vi "使用范例_多列数据存储.vi"() -> ()   [LabVIEW 2020]
panel:
  in  "y2":dbl[](array[numeric])=[1.0, 0.9951847266721969, 0.9807852804032304, 0.9569403357322088, 0.9238795325112867, 0.881921264348355, 0.8314696123025452, 0.773010453362737, 0.7071067811865476, 0.6343932841636455, 0.5555702330196023, 0.4713967368259978, 0.38268343236508984, 0.29028467725446233, 0.19509032201612833, 0.09801714032956077, 6.123233995736766e-17, -0.09801714032956065, -0.1950903220161282, -0.29028467725446216, -0.3826834323650897, -0.4713967368259977, -0.555570233019602, -0.6343932841636454, -0.7071067811865475, -0.773010453362737, -0.8314696123025453, -0.8819212643483549, -0.9238795325112867, -0.9569403357322088, -0.9807852804032304, -0.9951847266721968, -1.0, -0.9951847266721969, -0.9807852804032304, -0.9569403357322089, -0.9238795325112868, -0.881921264348355, -0.8314696123025455, -0.7730104533627371, -0.7071067811865477, -0.6343932841636459, -0.5555702330196022, -0.47139673682599786, -0.38268343236509034, -0.29028467725446244, -0.19509032201612866, -0.09801714032956045, -1.8369701987210297e-16, 0.09801714032956009, 0.1950903220161283, 0.29028467725446205, 0.38268343236509, 0.4713967368259976, 0.5555702330196018, 0.6343932841636456, 0.7071067811865474, 0.7730104533627367, 0.8314696123025452, 0.8819212643483548, 0.9238795325112865, 0.9569403357322088, 0.9807852804032303, 0.9951847266721969, 1.0]
  in  "x":dbl[](array[numeric])=[0.0, 0.09817477042468103, 0.19634954084936207, 0.2945243112740431, 0.39269908169872414, 0.4908738521234052, 0.5890486225480862, 0.6872233929727672, 0.7853981633974483, 0.8835729338221293, 0.9817477042468103, 1.0799224746714913, 1.1780972450961724, 1.2762720155208536, 1.3744467859455345, 1.4726215563702154, 1.5707963267948966, 1.6689710972195777, 1.7671458676442586, 1.8653206380689396, 1.9634954084936207, 2.061670178918302, 2.1598449493429825, 2.2580197197676637, 2.356194490192345, 2.454369260617026, 2.552544031041707, 2.650718801466388, 2.748893571891069, 2.84706834231575, 2.945243112740431, 3.043417883165112, 3.141592653589793, 3.2397674240144743, 3.3379421944391554, 3.436116964863836, 3.5342917352885173, 3.6324665057131984, 3.730641276137879, 3.8288160465625602, 3.9269908169872414, 4.025165587411922, 4.123340357836604, 4.221515128261284, 4.319689898685965, 4.417864669110647, 4.516039439535327, 4.614214209960009, 4.71238898038469, 4.81056375080937, 4.908738521234052, 5.006913291658733, 5.105088062083414, 5.203262832508095, 5.301437602932776, 5.399612373357457, 5.497787143782138, 5.595961914206819, 5.6941366846315, 5.792311455056181, 5.890486225480862, 5.988660995905543, 6.086835766330224, 6.1850105367549055, 6.283185307179586]
  in  "y1":dbl[](array[numeric])=[0.0, 0.0980171403295606, 0.19509032201612825, 0.29028467725446233, 0.3826834323650898, 0.47139673682599764, 0.5555702330196022, 0.6343932841636455, 0.7071067811865475, 0.773010453362737, 0.8314696123025452, 0.8819212643483549, 0.9238795325112867, 0.9569403357322089, 0.9807852804032304, 0.9951847266721968, 1.0, 0.9951847266721969, 0.9807852804032304, 0.9569403357322089, 0.9238795325112867, 0.881921264348355, 0.8314696123025455, 0.7730104533627371, 0.7071067811865476, 0.6343932841636455, 0.5555702330196022, 0.47139673682599786, 0.3826834323650899, 0.2902846772544624, 0.1950903220161286, 0.09801714032956083, 1.2246467991473532e-16, -0.09801714032956059, -0.19509032201612836, -0.2902846772544621, -0.38268343236508967, -0.47139673682599764, -0.555570233019602, -0.6343932841636453, -0.7071067811865475, -0.7730104533627367, -0.8314696123025452, -0.8819212643483549, -0.9238795325112865, -0.9569403357322088, -0.9807852804032303, -0.9951847266721969, -1.0, -0.9951847266721969, -0.9807852804032304, -0.9569403357322089, -0.9238795325112866, -0.881921264348355, -0.8314696123025455, -0.7730104533627369, -0.7071067811865477, -0.6343932841636459, -0.5555702330196022, -0.4713967368259979, -0.3826834323650904, -0.2902846772544625, -0.19509032201612872, -0.0980171403295605, -2.4492935982947064e-16]
  in  "文件头（最后一个字符是换行）":string="x y1 y2\n"
  in  "存储路径":path=path "D:/"
  in  "其他说明信息":string
  in  "测试项目":string="sin_cos"
  in  "样品名称":string="Math"
  in  "是否添加时间？":bool=TRUE
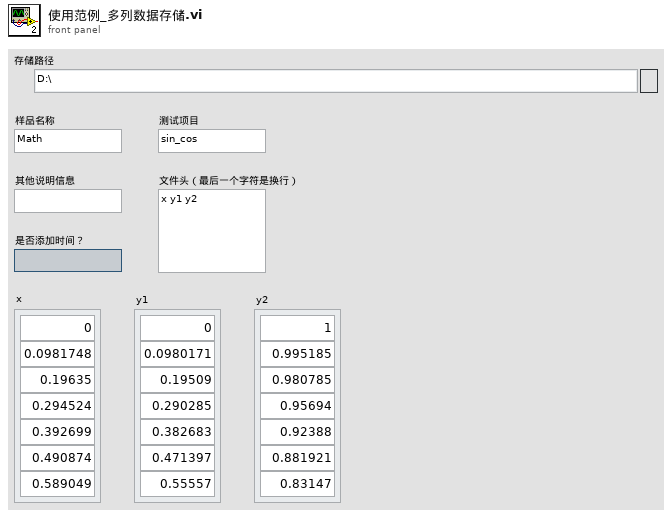
[diagram p1: front panel]
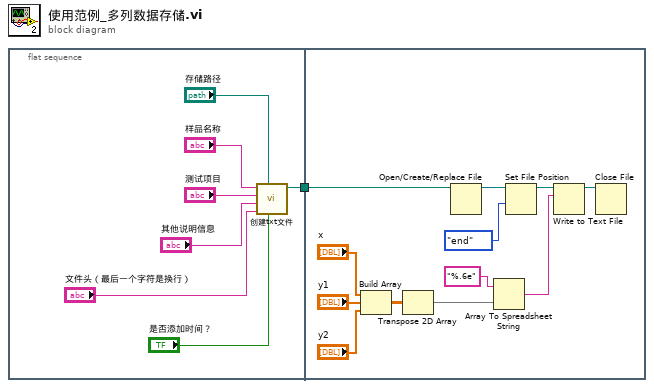
[diagram p0: block diagram]
diagram:
  n1 = flat-sequence {
    tunnel: [w2] -> w1
    tunnel: w1 -> [w10]
    frame #0 {
      n2 = call "创建txt文件.vi"("是否添加时间？"="是否添加时间？", "存储路径"="存储路径", "文件头（最后一个字符是换行）"="文件头（最后一个字符是换行）", "其他说明信息"="其他说明信息", "测试项目"="测试项目", "样品名称"="样品名称") -> ("文件路径"=w2:path)  [unwired: 5 in]
    }
    frame #1 {
      n3 = Build Array("x", "y1", "y2") -> (w17:dbl[][])
      n4 = Transpose 2D Array(2D array=w17) -> (transposed array=w16:dbl[][])
      n5 = Open/Create/Replace File(file path (use dialog)=w10) -> (refnum out=w12:refnum<file>)  [unwired: 5 in, 2 out]
      n6 = Array To Spreadsheet String(array=w16, 3:"%.6e" ("格式字符串")) -> (spreadsheet string=w9:string)  [unwired: 1 in]
      n7 = Set File Position(refnum=w12, from (0:start)=enum16{"start", "end", "current"}."end" ("自（0:起始）")) -> (refnum out=w13:refnum<file>)  [unwired: 2 in, 1 out]
      n8 = Write to Text File(file (use dialog)=w13, text=w9) -> (refnum out=w14:refnum<file>)  [unwired: 2 in, 2 out]
      n9 = Close File(refnum=w14) -> ()  [unwired: 1 in, 2 out]
    }
  }
